vi "ConfigureTrigger.vi"(8 "error in (no error)":errorcluster, 11 "Infiniium in":refnum<class "Infiniium.lvclass">) -> (0 "error out":errorcluster, 3 "Infiniium out":refnum<class "Infiniium.lvclass">)   [LabVIEW 2018, in "ScopePlugins.lvlib" / "Infiniium.lvclass"]
uses:
  Infiniium.lvclass
  Y:/Projects/PMUCal/Modules/Scope/ScopePlugins/ScopePluginBaseClass/ScopePluginsBase.lvclass
  ScopePluginBaseClass/ScopePluginsBase.lvclass/ScopePluginsBase.ctl
  ScopePluginBaseClass/Accessors/Read Handle.vi
  ScopePluginBaseClass/Accessors/Read Trigger.vi
  ScopePluginBaseClass/Accessors/Read Connected.vi
  <vilib>/Utility/error.llb/Error Cluster From Error Code.vi
  <instrlib>/Agilent 90000 Series/Public/Configure/Trigger/Configure Trigger (Edge).vi
  <instrlib>/Agilent 90000 Series/Public/Configure/Trigger/Configure Trigger (TV).vi
  <vilib>/ErrorRing/Error Ring.xnode
  <instrlib>/Agilent 90000 Series/Agilent 90000 Series.lvlib
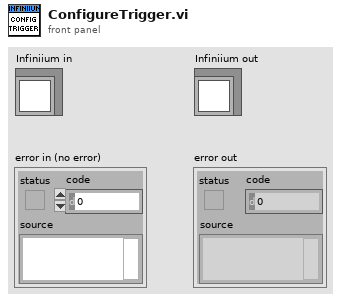
[diagram p1: front panel]
types:
  T1 = typedef "ScopePlugins.lvlib/Trigger.ctl" = cluster{"Coupling":enum16{"AC", "DC", "LF Reject", "HF Reject", "Noise Reject"}, "Holdoff":dbl, "Level":dbl, "Slope":enum16{"Negative", "Positive"}, "Source":string, "Type":enum16{"Edge", "Width", "Runt", "Glitch", "TV", "Immediate", "AC Line"}}
  T2 = enum16{"Edge", "Width", "Runt", "Glitch", "TV", "Immediate", "AC Line"}
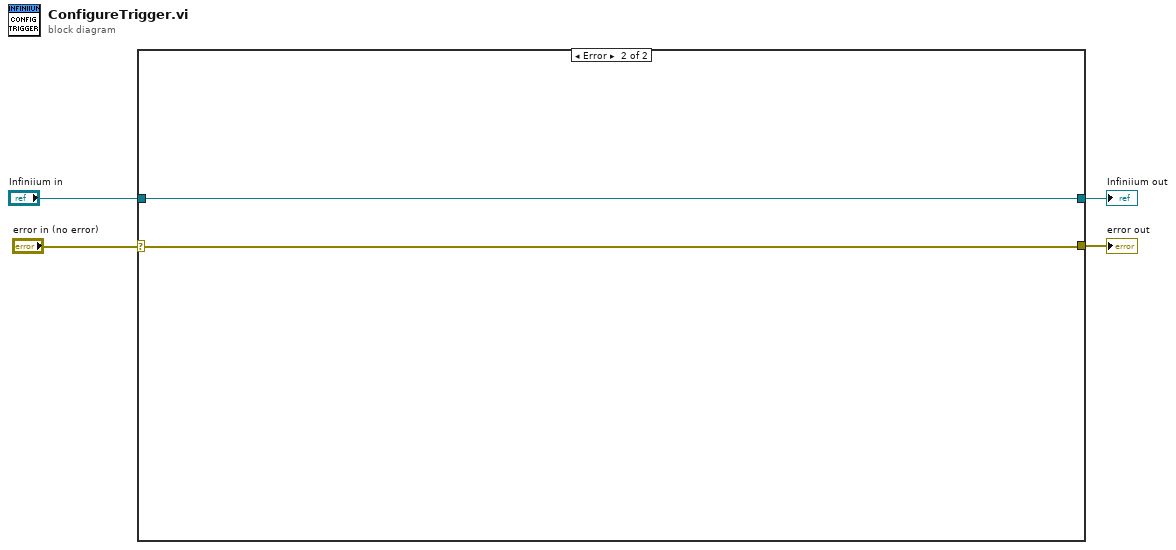
[diagram p0: block diagram]
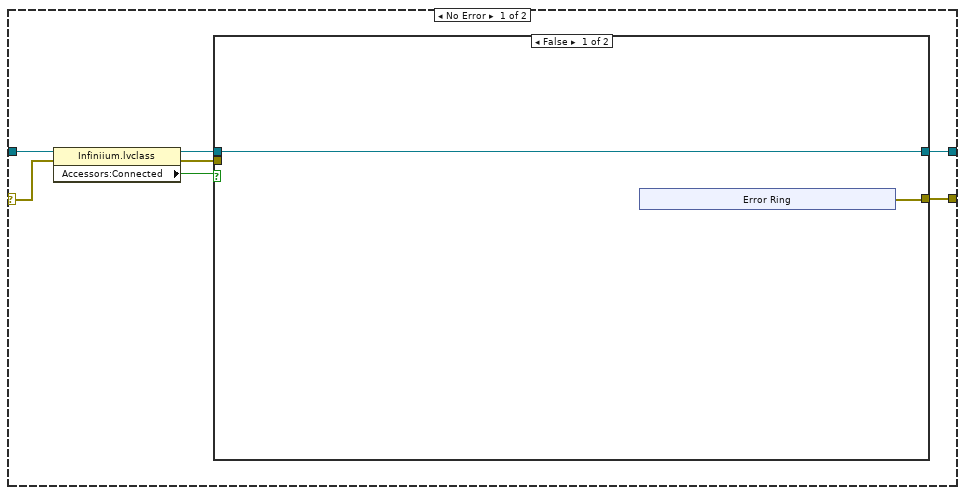
[diagram p2: hidden frame]
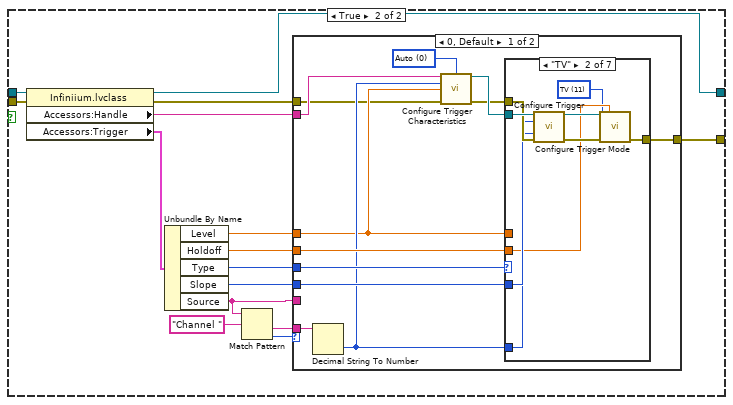
[diagram p3: hidden frame]
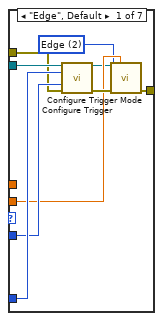
[diagram p4: hidden frame]
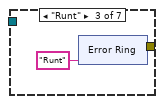
[diagram p5: hidden frame]
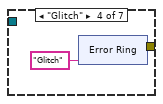
[diagram p6: hidden frame]
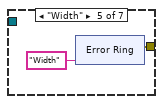
[diagram p7: hidden frame]
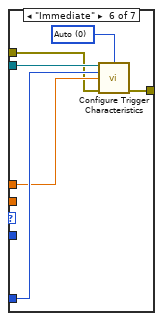
[diagram p8: hidden frame]
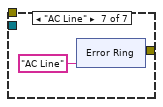
[diagram p9: hidden frame]
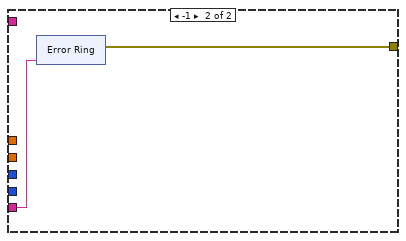
[diagram p10: hidden frame]
diagram:
  n1 = case shown="Error" "error in (no error)" {
    selector: "error in (no error)" -> [w10 w115]
    tunnel: "Infiniium in" -> [w11 w116]
    tunnel: [w6 w116] -> w2
    tunnel: [w5 w115] -> w1
    frame No Error {
      n2 = property class="Infiniium.lvclass"(reference=w11, error in=w10) -> (reference out=w8:refnum<class "Infiniium.lvclass">, error out=w7:errorcluster, "Accessors:Connected"=w9:bool)
      n3 = case shown="False" w9 {
        tunnel: w8 -> [w13 w33]
        tunnel: w7 -> [_ w32]
        tunnel: [w13 w20] -> w6
        tunnel: [w12 w19] -> w5
        frame False {
          n4 = xnode "Error Ring"() -> ("error out"=w12:errorcluster)
        }
        frame True {
          n5 = property class="Infiniium.lvclass"(reference=w33, error in=w32) -> (reference out=w20:refnum<class "Infiniium.lvclass">, error out=w24:errorcluster, "Accessors:Handle"=w26:string, "Accessors:Trigger"=w27:T1)
          n6 = Unbundle By Name(w27) -> ("Level"=w21:dbl, "Holdoff"=w22:dbl, "Type"=w23:T2, "Slope"=w25:enum16{"Negative", "Positive"}, "Source"=w29:string)
          n7 = Match Pattern(string=w29, regular expression="Channel ") -> (after substring=w28:string, offset past match=w30:i32)  [unwired: 1 in, 2 out]
          n8 = case shown="0, Default" w30 {
            tunnel: w29 -> [_ w107]
            tunnel: w28 -> [w45 _]
            tunnel: w26 -> [w40 _]
            tunnel: w25 -> [w44 _]
            tunnel: w24 -> [w35 _]
            tunnel: [w43 w106] -> w19
            tunnel: w23 -> [w42 _]
            tunnel: w22 -> [w41 _]
            tunnel: w21 -> [w36 _]
            frame 0, Default {
              w38 = 0 items=["Auto", "Triggered", "Single"] ("Sweep Mode (0: Auto)")
              n9 = Decimal String To Number(string=w45) -> (number=w37:i32)  [unwired: 2 in, 1 out]
              n10 = call <instrlib>:"Configure Trigger Characteristics.vi"("VISA resource name"=w40, "Sweep Mode (0: Auto)"=w38, "Trigger Source (1: Channel1)"=w37, "Trigger Level (0.0 V)"=w36, "error in (no error)"=w35) -> ("VISA resource name out"=w39:refnum<visa-resource-name>, "error out"=w34:errorcluster)  [unwired: 9 in]
              n11 = case shown="\"TV\"" w42 {
                tunnel: w39 -> [w54 w63 _ _ _ w94 _]
                tunnel: w37 -> [w53 w60 _ _ _ w93 _]
                tunnel: w44 -> [w52 w61 _ _ _ _ _]
                tunnel: w34 -> [w51 w62 _ _ _ w91 _]
                tunnel: [w46 w55 w65 w73 w82 w96 w98] -> w43
                tunnel: w41 -> [w49 w57 _ _ _ _ _]
                tunnel: w36 -> [_ _ _ _ _ w92 _]
                frame "Edge", Default {
                  w47 = 2 items=["Communication", "Delay", "Edge ", "Glitch", "Pattern", "Pulse Width ", "Runt", "Setup and Hold Time", "State", "Timeout", "Transition", "TV", "Window", "Advanced", "Serial Bus 1", "Serial Bus 2", "Serial Bus 3", "Serial Bus 4"] ("Trigger Mode (2: Edge)")
                  n12 = call-poly <instrlib>:"Configure Trigger.vi"("VISA resource name"=w54, "Trigger Source (1: Channel1)"=w53, "Edge Trigger Slope (0: Negative)"=w52, "error in (no error)"=w51) -> ("VISA resource name out"=w48:refnum<visa-resource-name>, "error out"=w50:errorcluster)  [unwired: 10 in]
                  n13 = call <instrlib>:"Configure Trigger Mode.vi"("VISA resource name"=w48, "Trigger Holdoff (1E-7 s)"=w49, "Trigger Mode (2: Edge)"=w47, "error in (no error)"=w50) -> ("error out"=w46:errorcluster)  [unwired: 10 in, 1 out]
                }
                frame "TV" {
                  w56 = 11 items=["Communication", "Delay", "Edge ", "Glitch", "Pattern", "Pulse Width ", "Runt", "Setup and Hold Time", "State", "Timeout", "Transition", "TV", "Window", "Advanced", "Serial Bus 1", "Serial Bus 2", "Serial Bus 3", "Serial Bus 4"] ("Trigger Mode (2: Edge)")
                  n14 = call-poly <instrlib>:"Configure Trigger.vi"("VISA resource name"=w63, "Trigger Source (1: Channel1)"=w60, "Trigger Polarity (0: Negative)"=w61, "error in (no error)"=w62) -> ("VISA resource name out"=w58:refnum<visa-resource-name>, "error out"=w59:errorcluster)  [unwired: 10 in]
                  n15 = call <instrlib>:"Configure Trigger Mode.vi"("VISA resource name"=w58, "Trigger Holdoff (1E-7 s)"=w57, "Trigger Mode (2: Edge)"=w56, "error in (no error)"=w59) -> ("error out"=w55:errorcluster)  [unwired: 10 in, 1 out]
                }
                frame "Runt" {
                  n16 = xnode "Error Ring"("parameter 0"="Runt") -> ("error out"=w65:errorcluster)
                }
                frame "Glitch" {
                  n17 = xnode "Error Ring"("parameter 0"="Glitch") -> ("error out"=w73:errorcluster)
                }
                frame "Width" {
                  n18 = xnode "Error Ring"("parameter 0"="Width") -> ("error out"=w82:errorcluster)
                }
                frame "Immediate" {
                  w95 = 0 items=["Auto", "Triggered", "Single"] ("Sweep Mode (0: Auto)")
                  n19 = call <instrlib>:"Configure Trigger Characteristics.vi"("VISA resource name"=w94, "Sweep Mode (0: Auto)"=w95, "Trigger Source (1: Channel1)"=w93, "Trigger Level (0.0 V)"=w92, "error in (no error)"=w91) -> ("error out"=w96:errorcluster)  [unwired: 9 in, 1 out]
                }
                frame "AC Line" {
                  n20 = xnode "Error Ring"("parameter 0"="AC Line") -> ("error out"=w98:errorcluster)
                }
              }
            }
            frame -1 {
              n21 = xnode "Error Ring"("parameter 0"=w107) -> ("error out"=w106:errorcluster)
            }
          }
        }
      }
    }
    frame Error {
    }
  }
  "error out" <- w1
  "Infiniium out" <- w2
